vi "Get_commandsss.vi"(10 "Vertical Slide Switch":bool, 11 "Address":T2) -> (0 "Command":T1, 2 "CMDADDR string":string, 3 "CMDADDR":u64 format="%x")   [LabVIEW 2020]
uses:
  VNA-Addresses.ctl
  VNA-Commands.ctl
panel:
  out "Address 2":u16 format="%x"
  out "Command":u16 format="%x"
  out "x+y":u16
  out "y":T1
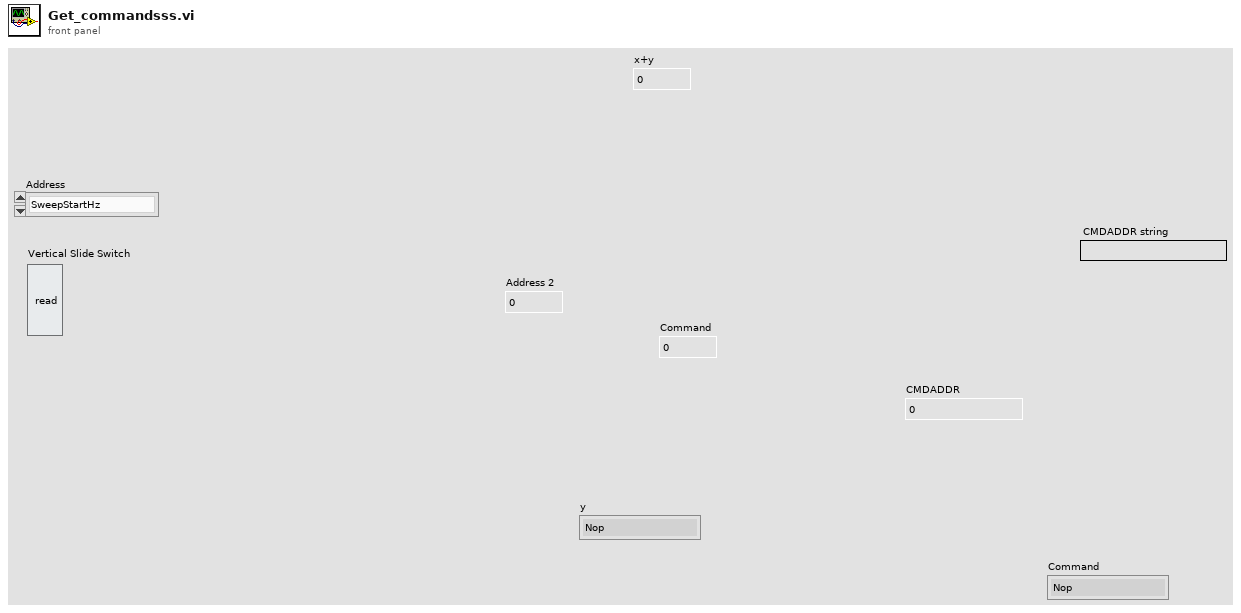
[diagram p1: front panel]
types:
  T1 = typedef "VNA-Commands.ctl" = enum16{"Nop", "Indicate", "Read 1B", "Read 2B", "Read 4B", "Read 8B", "Read FIFO", "Write 1B", "Write 2B", "Write 4B", "Write 8B", "Write FIFO"}
  T2 = typedef "VNA-Addresses.ctl" = enum16{"SweepStartHz", "SweepStopHz", "SweepPoints", "valuesPerFrequency", "RawSamplesMode", "ValuesFIFO", "deviceVariant", "protocolVersion", "hardwareRevision", "firmwareMajor", "firmwareMinor"}
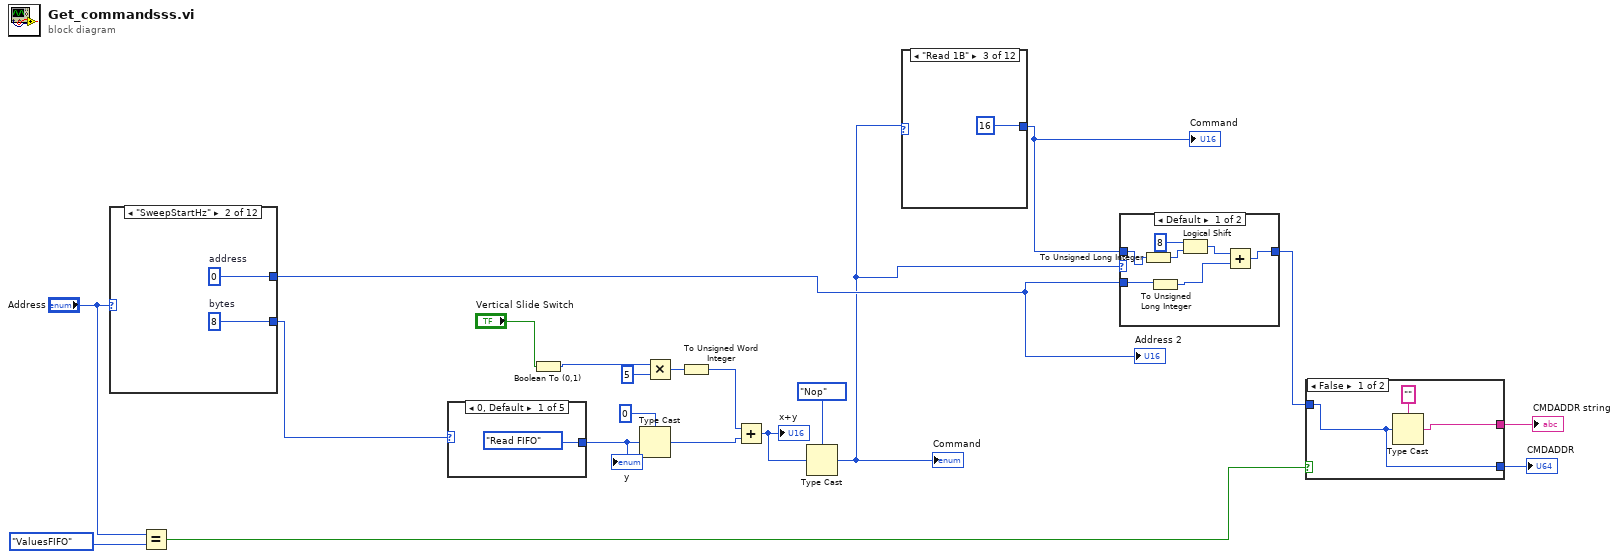
[diagram p0: block diagram]
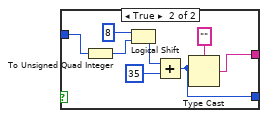
[diagram p2: hidden frame]
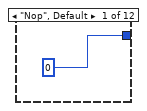
[diagram p3: hidden frame]
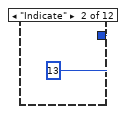
[diagram p4: hidden frame]
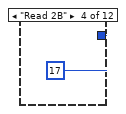
[diagram p5: hidden frame]
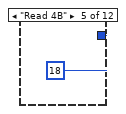
[diagram p6: hidden frame]
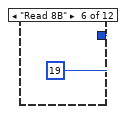
[diagram p7: hidden frame]
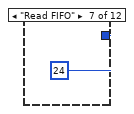
[diagram p8: hidden frame]
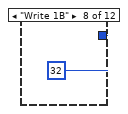
[diagram p9: hidden frame]
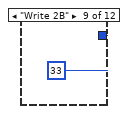
[diagram p10: hidden frame]
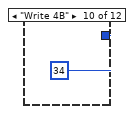
[diagram p11: hidden frame]
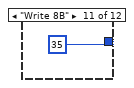
[diagram p12: hidden frame]
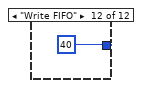
[diagram p13: hidden frame]
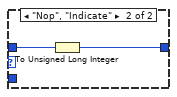
[diagram p14: hidden frame]
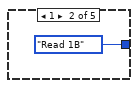
[diagram p15: hidden frame]
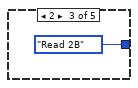
[diagram p16: hidden frame]
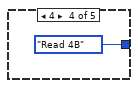
[diagram p17: hidden frame]
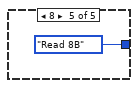
[diagram p18: hidden frame]
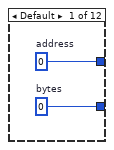
[diagram p19: hidden frame]
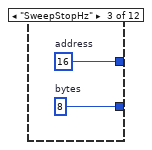
[diagram p20: hidden frame]
diagram:
  n1 = case shown="\"SweepStartHz\"" "Address" {
    tunnel: [w22 w24 w26 w28 w30 w32 w34 w36 w38 w40 w42 w44] -> w8
    tunnel: [w21 w23 w25 w27 w29 w31 w33 w35 w37 w39 w41 w43] -> w20
    frame Default {
      w21 = 0  # bytes
      w22 = u16 0  # address
    }
    frame "SweepStartHz" {
      w23 = 8  # bytes
      w24 = u16 0  # address
    }
    frame "SweepStopHz" {
      w25 = 8  # bytes
      w26 = u16 16  # address
    }
    frame "SweepPoints" {
      w27 = 2  # bytes
      w28 = u16 32  # address
    }
    frame "valuesPerFrequency" {
      w29 = 2  # bytes
      w30 = u16 34  # address
    }
    frame "RawSamplesMode" {
      w31 = 1  # bytes
      w32 = u16 38  # address
    }
    frame "ValuesFIFO" {
      w33 = 35  # bytes
      w34 = u16 48  # address
    }
    frame "deviceVariant" {
      w35 = 1  # bytes
      w36 = u16 240  # address
    }
    frame "protocolVersion" {
      w37 = 1  # bytes
      w38 = u16 241  # address
    }
    frame "hardwareRevision" {
      w39 = 1  # bytes
      w40 = u16 242  # address
    }
    frame "firmwareMajor" {
      w41 = 1  # bytes
      w42 = u16 243  # address
    }
    frame "firmwareMinor" {
      w43 = 1  # bytes
      w44 = u16 244  # address
    }
  }
  "Address 2" <- w8
  n2 = Equal?(x="Address", y=VNA-Addresses."ValuesFIFO") -> (x = y?=w2:bool)
  n3 = case shown="0, Default" w20 {
    tunnel: [VNA-Commands."Read FIFO" ("y") VNA-Commands."Read 1B" ("y") VNA-Commands."Read 2B" ("y") VNA-Commands."Read 4B" ("y") VNA-Commands."Read 8B" ("y")] -> w19
    frame 0, Default {
    }
    frame 1 {
    }
    frame 2 {
    }
    frame 4 {
    }
    frame 8 {
    }
  }
  "y" <- w19
  n4 = Boolean To (0,1)(Boolean="Vertical Slide Switch") -> (0, 1=w16:i16)
  n5 = Type Cast(type=u16 0, x=w19) -> (*(type *) &x=w11:u16)
  n6 = Multiply(x=w16, y=i16 5) -> (x*y=w14:i16)
  n7 = To Unsigned Word Integer(number=w14) -> (unsigned 16bit integer=w12:u16)
  n8 = Add(x=w12, y=w11) -> (x+y=w10:u16)
  "x+y" <- w10
  n9 = Type Cast(type=VNA-Commands."Nop" ("y"), x=w10) -> (*(type *) &x=w7:T1)
  "Command" <- w7
  n10 = case shown="\"Read 1B\"" w7 {
    tunnel: [u16 0 u16 13 u16 16 u16 17 u16 18 u16 19 u16 24 u16 32 u16 33 u16 34 u16 35 u16 40] -> w9
    frame "Nop", Default {
    }
    frame "Indicate" {
    }
    frame "Read 1B" {
    }
    frame "Read 2B" {
    }
    frame "Read 4B" {
    }
    frame "Read 8B" {
    }
    frame "Read FIFO" {
    }
    frame "Write 1B" {
    }
    frame "Write 2B" {
    }
    frame "Write 4B" {
    }
    frame "Write 8B" {
    }
    frame "Write FIFO" {
    }
  }
  "Command" <- w9
  n11 = case shown="Default" w7 {
    tunnel: w9 -> [w66 w70]
    tunnel: w8 -> [w63 _]
    tunnel: [w64 w69] -> w4
    frame Default {
      n12 = To Unsigned Long Integer(number=w66) -> (unsigned 32bit integer=w67:u32)
      n13 = To Unsigned Long Integer(number=w63) -> (unsigned 32bit integer=w62:u32)
      n14 = Logical Shift(y=i16 8, x=w67) -> (x << y=w65:u32)
      n15 = Add(x=w65, y=w62) -> (x+y=w64:u32)
    }
    frame "Nop", "Indicate" {
      n16 = To Unsigned Long Integer(number=w70) -> (unsigned 32bit integer=w69:u32)
    }
  }
  n17 = case shown="False" w2 {
    tunnel: w4 -> [w71 w79]
    tunnel: [w72 w75] -> w3
    tunnel: [w71 w74] -> w1
    frame False {
      n18 = Type Cast(type="", x=w71) -> (*(type *) &x=w72:string)
    }
    frame True {
      n19 = To Unsigned Quad Integer(1:w79) -> (0:w80:u64)
      n20 = Logical Shift(y=i16 8, x=w80) -> (x << y=w78:u64)
      n21 = Add(x=w78, y=u64 35) -> (x+y=w74:u64)
      n22 = Type Cast(type="", x=w74) -> (*(type *) &x=w75:string)
    }
  }
  "CMDADDR string" <- w3
  "CMDADDR" <- w1
